vi "WS1050 Bench CAP Characterization_Ver1.1.vi"() -> ()   [LabVIEW 2012]
panel:
  in  "Tab Control":enum32{"CONTROL", "INDICATION"}(tab)
  in  "RFFE Com Port":refnum<visa-resource-name>="COM3"
  in  "AD7747 Com Port":refnum<visa-resource-name>="COM1"
  in  "Init":bool=TRUE
  in  "Wafer":string="WS1050"
  in  "Lot":string="Toggle 7"
  in  "SN":string="01"
  in  "Temperature":string="RT"
  in  "Delay(ms)":u32=100
  in  "TMN DC\\CAP Data Log File Path":path=path "C:/Andy Tr/Temp"
  in  "String":string="WS1050 BENCH CAP CHARACTERIZATION Ver1.1"
  out "C3Cal (pF)":dbl=-4.9974111328125
  out "C1Cal (pF)":dbl=-4.5642919921875
  out "C2Cal (pF)":dbl=-4.9191376953125
  out "S_ValueC3(pF)":dbl=-4.9974111328125
  out "S_ValueC1(pF)":dbl=-4.5642919921875
  out "S_ValueC2(pF)":dbl=-4.9191376953125
  in  "Calib Socket":bool
  out "C1_Mesa(pF)":dbl
  out "C2_Mesa(pF)":dbl
  out "C3_Mesa(pF)":dbl
  in  "A364X_VDD":refnum<visa-resource-name>="GPIB1::6::INSTR"
  in  "IDD Limit":dbl=0.02 format="%.2p"
  in  "VDD":dbl=3.3
  in  "CP Setting":i32(ring) items=["CP OFF", "CP ON", "DVA OFF", "DVA ON", "ECAL OFF", "ECAL ON", "CP 40.25V", "CP 35V", "CP 38V", "CP 44V", "CP 50V", "CP 23.75V", "CP 25.25V", "CP 29.75V", "C1 ON", "C1 OFF", "C2 ON", "C2 OFF", "C3 ON", "C3 OFF"]
  in  "Send":bool
  in  "Init AD7747":bool
  in  "Keithley 2000":refnum<visa-resource-name>
  out "C_min(pF)":string[](array[string])
  out "C_Max":string[](array[string])
  out "C_Min2(pF)":string[](array[string])
  out "error out":errorcluster
  in  "error in (no error)":errorcluster
  in  "stop":bool
  in  "Abort":bool
  in  "Start Test":bool
  out "Running loop":i32
  # "Company:  WiSpry Inc\n198 Fairbanks Ste 198 Irvine\n\nCreated by:  Andy V Tran\nDate:  03/11/2015\nTP:  WS1050 Bench\nCAP Characterization"
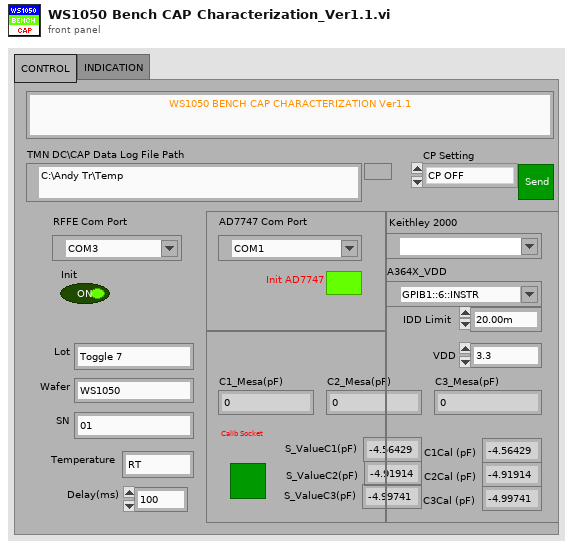
[diagram p1: front panel]
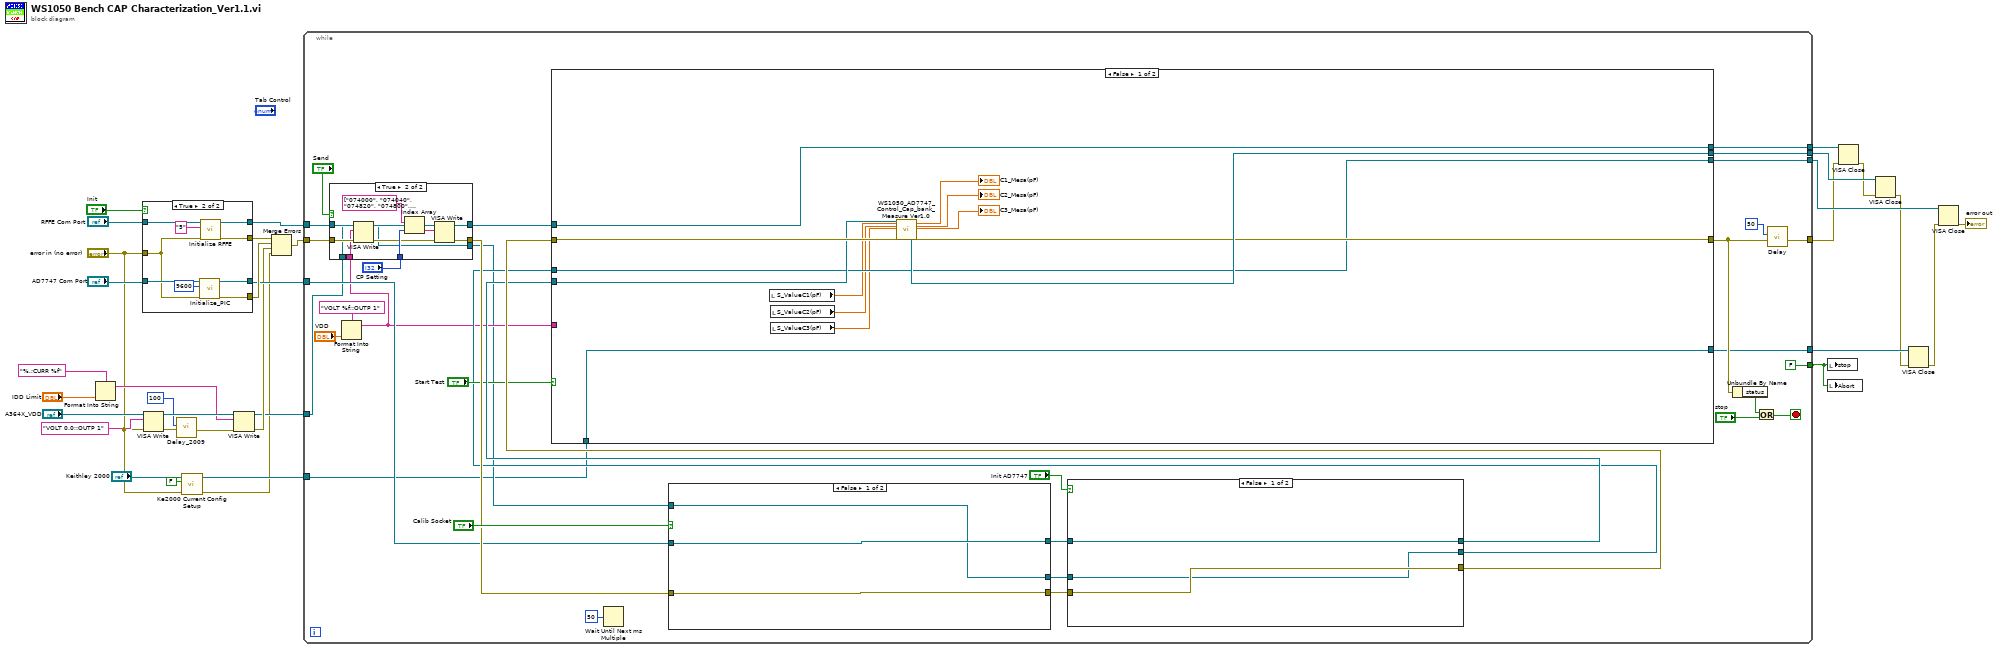
[diagram p0: block diagram]
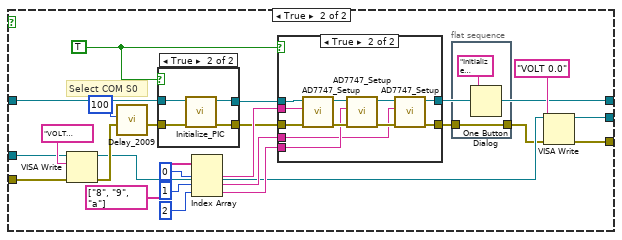
[diagram p3: hidden frame]
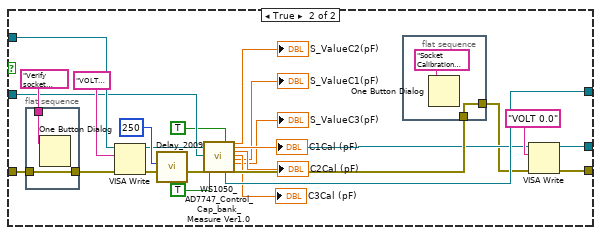
[diagram p6: hidden frame]
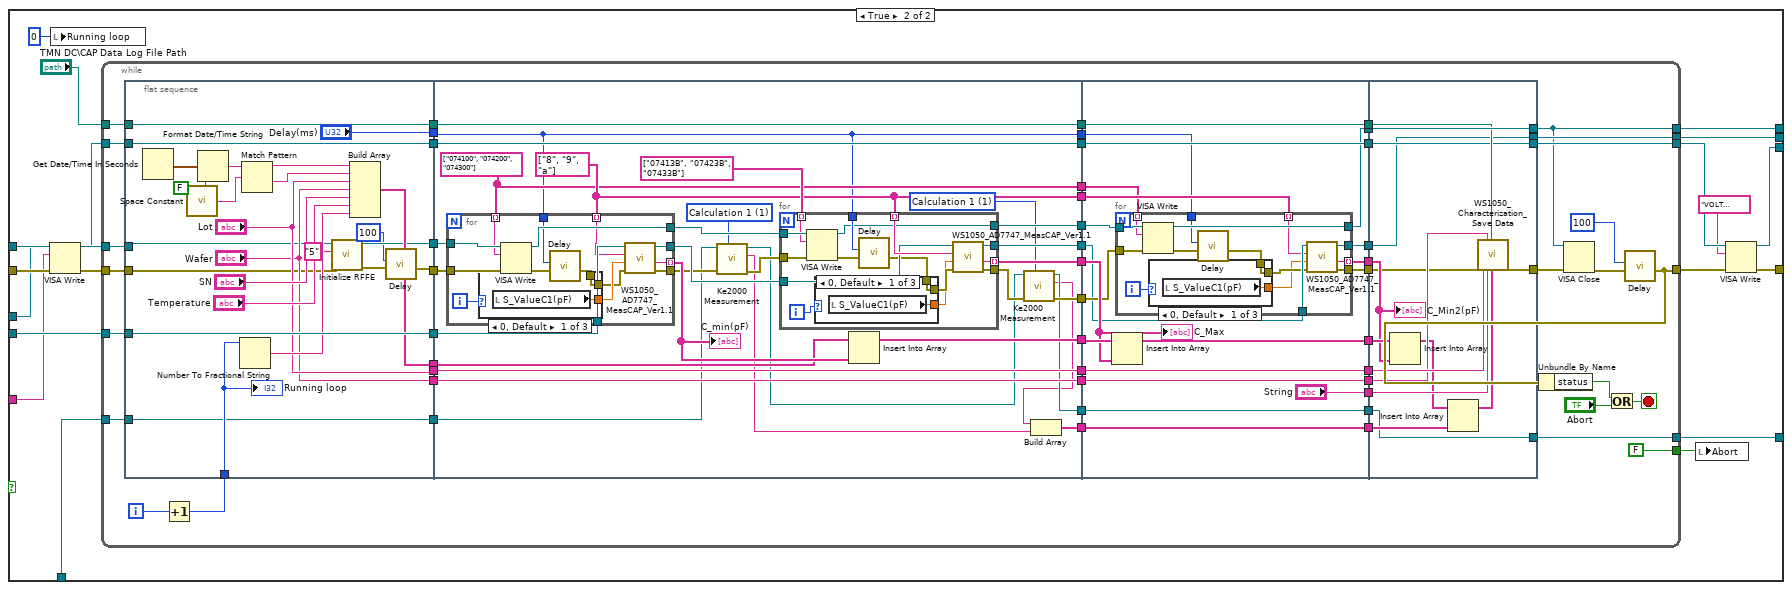
[diagram p7: hidden frame]
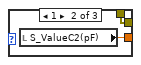
[diagram p8: hidden frame]
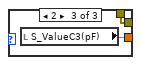
[diagram p9: hidden frame]
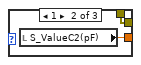
[diagram p10: hidden frame]
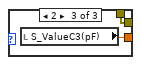
[diagram p11: hidden frame]
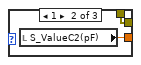
[diagram p12: hidden frame]
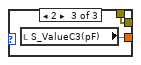
[diagram p13: hidden frame]
diagram:
  n1 = Format Into String(format string="%.;CURR %f", "IDD Limit") -> (resulting string=w24:string)  [unwired: 2 in, 1 out]
  n2 = case shown="True" "Init" {
    tunnel: "RFFE Com Port" -> [w37 w46]
    tunnel: [w37 w44] -> w33
    tunnel: "AD7747 Com Port" -> [w35 w42]
    tunnel: [w36 w41] -> w31
    tunnel: [w36 w40] -> w30
    tunnel: [w35 w39] -> w28
    tunnel: "error in (no error)" -> [w36 w38]
    frame False {
    }
    frame True {
      n3 = call "Initialize_PIC.vi"("error in (no error)"=w38, "baud rate"=u32 9600, "Select Com Port"=w42) -> ("error out"=w40:errorcluster, "VISA resource name out"=w39:refnum<visa-resource-name>)  [unwired: 7 in]
      n4 = call "Initialize RFFE.vi"("error in (no error)"=w38, "write buffer"="5", "Select Com Port"=w46) -> ("error out"=w41:errorcluster, "VISA resource name out"=w44:refnum<visa-resource-name>)  [unwired: 7 in]
    }
  }
  n5 = VISA Write(VISA resource name="A364X_VDD", write buffer="VOLT 0.0;:OUTP 1", error in (no error)="error in (no error)") -> (VISA resource name out=w25:refnum<visa-resource-name>, error out=w21:errorcluster)  [unwired: 1 out]
  n6 = call "Delay_2009.vi"("error in (no error)"=w21, "milliseconds to wait"=u32 100) -> ("error out"=w26:errorcluster)  [unwired: 9 in]
  n7 = call "Ke2000 Current Config Setup.vi"("error in (no error)"="error in (no error)", "Auto Range(T/F)"=FALSE, "VISA resource name"="Keithley 2000") -> ("error out"=w4:errorcluster, "VISA resource name out"=w5:refnum<visa-resource-name>)  [unwired: 7 in]
  n8 = VISA Write(VISA resource name=w25, write buffer=w24, error in (no error)=w26) -> (VISA resource name out=w16:refnum<visa-resource-name>, error out=w17:errorcluster)  [unwired: 1 out]
  n9 = Merge Errors(w31, w30, w17, w4) -> (w29:errorcluster)
  n10 = while {
    tunnel: w33 -> [w77]
    tunnel: w29 -> [w78]
    tunnel: w28 -> [w65]
    tunnel: [w73] -> w12
    tunnel: [w71] -> w15
    tunnel: [w70] -> w14
    tunnel: w16 -> [w52]
    tunnel: [w56] -> w13
    tunnel: [FALSE ("stop")] -> w9
    tunnel: w5 -> [w48]
    tunnel: [w47] -> w3
    stop <- w68 stop-if-true
    n11 = Format Into String(format string="VOLT %f;:OUTP 1", "VDD") -> (resulting string=w51:string)  [unwired: 2 in, 1 out]
    n12 = case shown="True" "Send" {
      tunnel: w78 -> [w404 w410]
      tunnel: [w404 w414] -> w66
      tunnel: [w403 w413] -> w76
      tunnel: "CP Setting" -> [_ w412]
      tunnel: w77 -> [w403 w411]
      tunnel: w52 -> [w402 w409]
      tunnel: w51 -> [_ w408]
      tunnel: [w402 w406] -> w50
      frame False {
      }
      frame True {
        n13 = VISA Write(VISA resource name=w409, write buffer=w408, error in (no error)=w410) -> (VISA resource name out=w406:refnum<visa-resource-name>, error out=w407:errorcluster)  [unwired: 1 out]
        n14 = Index Array(array=string[] ["074000", "074040", "074820", "074800", "074044", "074040", "074776", "07476F", "074773", "07477B", "07477C", "074760", "074762", "074768", "07413B", "074100", "07423B", "074200", "07433B", "074300"], index=w412) -> (element=w415:string)
        n15 = VISA Write(VISA resource name=w411, write buffer=w415, error in (no error)=w407) -> (VISA resource name out=w413:refnum<visa-resource-name>, error out=w414:errorcluster)  [unwired: 1 out]
      }
    }
    n16 = Wait Until Next ms Multiple(millisecond multiple=u32 50) -> ()  [unwired: 1 out]
    n17 = case shown="False" "Calib Socket" {
      tunnel: w66 -> [w131 w154]
      tunnel: [w131 w137] -> w60
      tunnel: w65 -> [w130 w135]
      tunnel: w50 -> [w129 w143]
      tunnel: [w129 w138] -> w61
      tunnel: [w130 w152] -> w59
      frame False {
      }
      frame True {
        n18 = flat-sequence {
          tunnel: [w157] -> w144
          tunnel: w154 -> [w157]
          tunnel: "Verify socket should be empty" ("message") -> [w156]
          frame #0 {
            n19 = One Button Dialog(message=w156) -> ()  [unwired: 1 in, 1 out]
          }
        }
        n20 = VISA Write(VISA resource name=w143, write buffer="VOLT 3.3;:OUTP 1", error in (no error)=w144) -> (VISA resource name out=w139:refnum<visa-resource-name>, error out=w141:errorcluster)  [unwired: 1 out]
        n21 = call "Delay_2009.vi"("error in (no error)"=w141, "milliseconds to wait"=u32 250) -> ("error out"=w134:errorcluster)  [unwired: 9 in]
        n22 = call "WS1050_AD7747_Control_Cap_bank_Measure Ver1.0.vi"("Select Com Port"=w135, "errorin"=w134, "Push Button to Measue Cap"=TRUE, "Push Button to Calibrate"=TRUE ("Push Button to Initialize AD7747")) -> ("Com Port Out"=w152:refnum<visa-resource-name>, "C2(pF)"=→"S_ValueC2(pF)":dbl, "C1_Mesa(pF)"=→"C1Cal (pF)":dbl, "C2_Mesa(pF)"=→"C2Cal (pF)":dbl, "C3_Mesa(pF)"=→"C3Cal (pF)":dbl, "C1(pF)"=→"S_ValueC1(pF)":dbl, "C3(pF)"=→"S_ValueC3(pF)":dbl, "error out"=w153:errorcluster)  [unwired: 16 in]
        n23 = flat-sequence {
          tunnel: [w158] -> w136
          tunnel: w153 -> [w158]
          frame #0 {
            n24 = One Button Dialog(message="Socket Calibration Completed, Please insert DUT into the Socket") -> ()  [unwired: 1 in, 1 out]
          }
        }
        n25 = VISA Write(VISA resource name=w139, write buffer="VOLT 0.0", error in (no error)=w136) -> (VISA resource name out=w138:refnum<visa-resource-name>, error out=w137:errorcluster)  [unwired: 1 out]
      }
    }
    n26 = case shown="False" "Init AD7747" {
      tunnel: w59 -> [w82 w107]
      tunnel: [w83 w87] -> w63
      tunnel: w60 -> [w83 w92]
      tunnel: [w82 w85] -> w62
      tunnel: w61 -> [w81 w93]
      tunnel: [w81 w88] -> w57
      frame False {
      }
      frame True {
        w97 = TRUE
        # "Select COM S0"
        n27 = VISA Write(VISA resource name=w93, write buffer="VOLT 3.3;:OUTP 1", error in (no error)=w92) -> (VISA resource name out=w89:refnum<visa-resource-name>, error out=w91:errorcluster)  [unwired: 1 out]
        n28 = call "Delay_2009.vi"("error in (no error)"=w91, "milliseconds to wait"=u32 100) -> ("error out"=w95:errorcluster)  [unwired: 9 in]
        n29 = case shown="True" w97 {
          tunnel: [w121 w126] -> w98
          tunnel: [w122 w125] -> w106
          tunnel: w107 -> [w122 w124]
          tunnel: w95 -> [w121 w123]
          frame False {
          }
          frame True {
            n30 = call "Initialize_PIC.vi"("error in (no error)"=w123, "Select Com Port"=w124) -> ("error out"=w126:errorcluster, "VISA resource name out"=w125:refnum<visa-resource-name>)  [unwired: 8 in]
          }
        }
        n31 = Index Array(array=string[] ["8", "9", "a"], index #1=0 ("index"), index #2=1 ("index"), index #3=2 ("index")) -> (element #1=w101:string, element #2=w100:string, element #3=w99:string)
        n32 = case shown="True" w97 {
          tunnel: w98 -> [w109 w112]
          tunnel: [w109 w110] -> w84
          tunnel: w106 -> [w108 w120]
          tunnel: w101 -> [_ w115]
          tunnel: w99 -> [_ w114]
          tunnel: w100 -> [_ w113]
          tunnel: [w108 w111] -> w85
          frame False {
          }
          frame True {
            n33 = call "AD7747_Setup.vi"("error in"=w112, "AD7747_Number"=w115, "Control"=w120) -> ("error out"=w119:errorcluster, "Control out"=w118:refnum<visa-resource-name>)  [unwired: 6 in, 1 out]
            n34 = call "AD7747_Setup.vi"("error in"=w119, "AD7747_Number"=w114, "Control"=w118) -> ("error out"=w117:errorcluster, "Control out"=w116:refnum<visa-resource-name>)  [unwired: 6 in, 1 out]
            n35 = call "AD7747_Setup.vi"("error in"=w117, "AD7747_Number"=w113, "Control"=w116) -> ("error out"=w110:errorcluster, "Control out"=w111:refnum<visa-resource-name>)  [unwired: 6 in, 1 out]
          }
        }
        n36 = flat-sequence {
          tunnel: w84 -> [w127]
          tunnel: [w127] -> w86
          frame #0 {
            n37 = One Button Dialog(message="Initialize AD7747 completed!") -> ()  [unwired: 1 in, 1 out]
          }
        }
        n38 = VISA Write(VISA resource name=w89, write buffer="VOLT 0.0", error in (no error)=w86) -> (VISA resource name out=w88:refnum<visa-resource-name>, error out=w87:errorcluster)  [unwired: 1 out]
      }
    }
    n39 = case shown="False" "Start Test" {
      tunnel: w76 -> [w165 w191]
      tunnel: w63 -> [w172 w186]
      tunnel: w62 -> [w171 w190]
      tunnel: [w169 w184] -> w74
      tunnel: [w165 w189] -> w71
      tunnel: [w170 w188] -> w70
      tunnel: w57 -> [w164 w185]
      tunnel: [w164 w181] -> w56
      tunnel: w51 -> [_ w176]
      tunnel: w48 -> [w160 w174]
      tunnel: [w160 w173] -> w47
      frame False {
        n40 = local read "S_ValueC1(pF)"() -> (w163:dbl)
        n41 = local read "S_ValueC2(pF)"() -> (w162:dbl)
        n42 = local read "S_ValueC3(pF)"() -> (w161:dbl)
        n43 = call "WS1050_AD7747_Control_Cap_bank_Measure Ver1.0.vi"("Select Com Port"=w171, "S_Value C1"=w163, "S_Value C2"=w162, "S_Value C3"=w161, "errorin"=w172) -> ("Com Port Out"=w170:refnum<visa-resource-name>, "C1_Mesa(pF)"=→"C1_Mesa(pF)":dbl, "C2_Mesa(pF)"=→"C2_Mesa(pF)":dbl, "C3_Mesa(pF)"=→"C3_Mesa(pF)":dbl, "error out"=w169:errorcluster)  [unwired: 15 in, 3 out]
      }
      frame True {
        n44 = VISA Write(VISA resource name=w185, write buffer=w176, error in (no error)=w186) -> (VISA resource name out=w183:refnum<visa-resource-name>, error out=w187:errorcluster)  [unwired: 1 out]
        n45 = local write "Running loop"(0 ("Loop Running")) -> ()
        n46 = while {
          tunnel: w191 -> [w244]
          tunnel: w187 -> [w243]
          tunnel: w190 -> [w242]
          tunnel: [w199] -> w180
          tunnel: "TMN DC\\CAP Data Log File Path" -> [w236]
          tunnel: [w202] -> w189
          tunnel: [w232] -> w188
          tunnel: w183 -> [w228]
          tunnel: [w225] -> w182
          tunnel: [FALSE ("Abort")] -> w177
          tunnel: w174 -> [w198]
          tunnel: [w192] -> w173
          i -> [w219]
          stop <- w239 stop-if-true
          n47 = flat-sequence {
            tunnel: w228 -> [w270]
            tunnel: w236 -> [w271]
            tunnel: w242 -> [w272]
            tunnel: w243 -> [w253]
            tunnel: w244 -> [w254]
            tunnel: [w250] -> w217
            tunnel: [w251] -> w216
            tunnel: [w272] -> w215
            tunnel: [w271] -> w214
            tunnel: [w270] -> w213
            tunnel: w212 -> [w257]
            tunnel: [w260] -> w211
            tunnel: ["Lot"] -> w210
            tunnel: ["Wafer"] -> w207
            tunnel: ["Delay(ms)"] -> w203
            tunnel: w198 -> [w248]
            tunnel: [w248] -> w197
            tunnel: [w292] -> w247
            tunnel: [w297] -> w246
            tunnel: [w279] -> w241
            tunnel: [w296] -> w235
            tunnel: [w295] -> w233
            tunnel: [w294] -> w230
            tunnel: [w291] -> w226
            tunnel: [w290] -> w224
            tunnel: [w285] -> w223
            tunnel: [w289] -> w222
            tunnel: w217 -> [w303]
            tunnel: w216 -> [w302]
            tunnel: w215 -> [w299]
            tunnel: w214 -> [w294]
            tunnel: w213 -> [w291]
            tunnel: w211 -> [w288]
            tunnel: w210 -> [w287]
            tunnel: [w287] -> w209
            tunnel: w207 -> [w286]
            tunnel: [w286] -> w206
            tunnel: w203 -> [w285]
            tunnel: w197 -> [w282]
            tunnel: [w277] -> w196
            tunnel: [w273] -> w194
            tunnel: w247 -> [w365]
            tunnel: w246 -> [w364]
            tunnel: [w363] -> w245
            tunnel: w241 -> [w359]
            tunnel: [w360] -> w240
            tunnel: w235 -> [w355]
            tunnel: [w354] -> w234
            tunnel: w233 -> [w353]
            tunnel: [w362] -> w231
            tunnel: w230 -> [w362]
            tunnel: [w361] -> w227
            tunnel: w226 -> [w361]
            tunnel: w224 -> [w358]
            tunnel: w223 -> [w357]
            tunnel: w222 -> [w356]
            tunnel: [w352] -> w221
            tunnel: [w351] -> w220
            tunnel: w209 -> [w350]
            tunnel: [w350] -> w208
            tunnel: w206 -> [w349]
            tunnel: [w349] -> w205
            tunnel: ["String"] -> w204
            tunnel: w196 -> [w347]
            tunnel: [w347] -> w195
            tunnel: w194 -> [w346]
            tunnel: [w346] -> w193
            tunnel: w245 -> [w396]
            tunnel: w240 -> [w391]
            tunnel: [w401] -> w201
            tunnel: w234 -> [w400]
            tunnel: [w400] -> w202
            tunnel: [w397] -> w232
            tunnel: w231 -> [w399]
            tunnel: w227 -> [w398]
            tunnel: [w398] -> w225
            tunnel: w221 -> [w397]
            tunnel: w220 -> [w395]
            tunnel: w208 -> [w394]
            tunnel: w205 -> [w393]
            tunnel: w204 -> [w392]
            tunnel: w195 -> [w387]
            tunnel: w193 -> [w389]
            tunnel: [w387] -> w192
            frame #0 {
              n48 = Get Date/Time In Seconds() -> (seconds since 1Jan1904=w266:timestamp)
              n49 = call <vilib>:"Space Constant.vi"() -> ("String"=w269:string)
              n50 = Format Date/Time String(seconds (now)=w266, UTC format=FALSE) -> (date/time string=w267:string)  [unwired: 1 out]
              n51 = Number To Fractional String(number=w257) -> (F-format string=w261:string)  [unwired: 3 in]
              n52 = Match Pattern(string=w267, regular expression=w269) -> (before substring=w265:string, after substring=w264:string)  [unwired: 3 out]
              n53 = call "Initialize RFFE.vi"("error in (no error)"=w253, "write buffer"="5", "Select Com Port"=w254) -> ("error out"=w252:errorcluster, "VISA resource name out"=w250:refnum<visa-resource-name>)  [unwired: 7 in]
              n54 = Build Array(w265, w264, "Lot", "Wafer", "SN", "Temperature", w261) -> (w260:string[])
              n55 = call "Delay.vi"("error in (no error)"=w252, "milliseconds to wait"=u32 100) -> ("error out"=w251:errorcluster)  [unwired: 9 in]
              "Running loop" <- w257
            }
            frame #1 {
              w276 = u16 1 items=["Function", "Calculation 1", "Calculation 2", "Calculation 3"] ("Source (0: Function)")
              w281 = u16 1 items=["Function", "Calculation 1", "Calculation 2", "Calculation 3"] ("Source (0: Function)")
              w290 = string[] ["8", "9", "a"]
              w289 = string[] ["074100", "074200", "074300"]
              n56 = for {
                tunnel: w303 -> [w339]
                tunnel: w302 -> [w338]
                tunnel: w289 -> [w337] mode=indexing
                tunnel: [w336] -> w300
                tunnel: w299 -> [w335]
                tunnel: [w334] -> w298
                tunnel: [w333] -> w283
                tunnel: w285 -> [w331]
                tunnel: w290 -> [w330] mode=indexing
                tunnel: [w329] -> w293 mode=indexing
                i -> [w328]
                n57 = VISA Write(VISA resource name=w339, write buffer=w337, error in (no error)=w338) -> (VISA resource name out=w336:refnum<visa-resource-name>, error out=w332:errorcluster)  [unwired: 1 out]
                n58 = call "Delay.vi"("error in (no error)"=w332, "milliseconds to wait"=w331) -> ("error out"=w326:errorcluster)  [unwired: 9 in]
                n59 = case shown="0, Default" w328 {
                  tunnel: [w341 w343 w345] -> w327
                  tunnel: w326 -> [w340 w342 w344]
                  tunnel: [w340 w342 w344] -> w325
                  frame 0, Default {
                    n60 = local read "S_ValueC1(pF)"() -> (w341:dbl)
                  }
                  frame 1 {
                    n61 = local read "S_ValueC2(pF)"() -> (w343:dbl)
                  }
                  frame 2 {
                    n62 = local read "S_ValueC3(pF)"() -> (w345:dbl)
                  }
                }
                n63 = call "WS1050_AD7747_MeasCAP_Ver1.1.vi"("error in (no error)"=w325, "OFFSet Cal"=w327, "AD7747_Number"=w330, "Control"=w335) -> ("error"=w333:errorcluster, "CAP (pF)"=w329:string, "Control out"=w334:refnum<visa-resource-name>)  [unwired: 4 in, 1 out]
              }
              "C_min(pF)" <- w293
              n64 = call "Ke2000 Measurement.vi"("Source (0: Function)"=w281, "error in (no error)"=w283, "VISA resource name"=w282) -> ("error out"=w284:errorcluster, "Meas in micro"=w274:string, "VISA resource name out"=w278:refnum<visa-resource-name>)  [unwired: 3 in, 3 out]
              n65 = for {
                tunnel: w300 -> [w318]
                tunnel: w284 -> [w317]
                tunnel: string[] ["07413B", "07423B", "07433B"] -> [w316] mode=indexing
                tunnel: w285 -> [w314]
                tunnel: w290 -> [w313] mode=indexing
                tunnel: [w312] -> w280
                tunnel: [w311] -> w295
                tunnel: [w310] -> w296
                tunnel: w298 -> [w309]
                tunnel: [w308] -> w297 mode=indexing
                i -> [w306]
                n66 = VISA Write(VISA resource name=w318, write buffer=w316, error in (no error)=w317) -> (VISA resource name out=w310:refnum<visa-resource-name>, error out=w315:errorcluster)  [unwired: 1 out]
                n67 = call "Delay.vi"("error in (no error)"=w315, "milliseconds to wait"=w314) -> ("error out"=w305:errorcluster)  [unwired: 9 in]
                n68 = case shown="0, Default" w306 {
                  tunnel: [w320 w322 w324] -> w304
                  tunnel: w305 -> [w319 w321 w323]
                  tunnel: [w319 w321 w323] -> w307
                  frame 0, Default {
                    n69 = local read "S_ValueC1(pF)"() -> (w320:dbl)
                  }
                  frame 1 {
                    n70 = local read "S_ValueC2(pF)"() -> (w322:dbl)
                  }
                  frame 2 {
                    n71 = local read "S_ValueC3(pF)"() -> (w324:dbl)
                  }
                }
                n72 = call "WS1050_AD7747_MeasCAP_Ver1.1.vi"("error in (no error)"=w307, "OFFSet Cal"=w304, "AD7747_Number"=w313, "Control"=w309) -> ("error"=w312:errorcluster, "CAP (pF)"=w308:string, "Control out"=w311:refnum<visa-resource-name>)  [unwired: 4 in, 1 out]
              }
              n73 = Insert Into Array(array=w288, new element=w293) -> (w292:string[])  [unwired: 1 in]
              n74 = call "Ke2000 Measurement.vi"("Source (0: Function)"=w276, "error in (no error)"=w280, "VISA resource name"=w278) -> ("error out"=w279:errorcluster, "Meas in micro"=w275:string, "VISA resource name out"=w277:refnum<visa-resource-name>)  [unwired: 3 in, 3 out]
              n75 = Build Array(w275, w274) -> (w273:string[])
            }
            frame #2 {
              n76 = Insert Into Array(array=w365, new element=w364) -> (w363:string[])  [unwired: 1 in]
              n77 = for {
                tunnel: w355 -> [w380]
                tunnel: w359 -> [w379]
                tunnel: w356 -> [w378] mode=indexing
                tunnel: [w377] -> w354
                tunnel: w353 -> [w376]
                tunnel: [w375] -> w352
                tunnel: [w374] -> w360
                tunnel: w357 -> [w372]
                tunnel: w358 -> [w371] mode=indexing
                tunnel: [w370] -> w351 mode=indexing
                i -> [w369]
                n78 = VISA Write(VISA resource name=w380, write buffer=w378, error in (no error)=w379) -> (VISA resource name out=w377:refnum<visa-resource-name>, error out=w373:errorcluster)  [unwired: 1 out]
                n79 = call "Delay.vi"("error in (no error)"=w373, "milliseconds to wait"=w372) -> ("error out"=w367:errorcluster)  [unwired: 9 in]
                n80 = case shown="0, Default" w369 {
                  tunnel: [w382 w384 w386] -> w366
                  tunnel: w367 -> [w381 w383 w385]
                  tunnel: [w381 w383 w385] -> w368
                  frame 0, Default {
                    n81 = local read "S_ValueC1(pF)"() -> (w382:dbl)
                  }
                  frame 1 {
                    n82 = local read "S_ValueC2(pF)"() -> (w384:dbl)
                  }
                  frame 2 {
                    n83 = local read "S_ValueC3(pF)"() -> (w386:dbl)
                  }
                }
                n84 = call "WS1050_AD7747_MeasCAP_Ver1.1.vi"("error in (no error)"=w368, "OFFSet Cal"=w366, "AD7747_Number"=w371, "Control"=w376) -> ("error"=w374:errorcluster, "CAP (pF)"=w370:string, "Control out"=w375:refnum<visa-resource-name>)  [unwired: 4 in, 1 out]
              }
              "C_Max" <- w364
            }
            frame #3 {
              n85 = Insert Into Array(array=w396, new element=w395) -> (w390:string[])  [unwired: 1 in]
              n86 = Insert Into Array(array=w390, new element=w389) -> (w388:string[])  [unwired: 1 in]
              n87 = call "WS1050_Characterization_Save Data.vi"("error in (no error)"=w391, "Lot"=w394, "Wafer"=w393, "TP"=w392, "TMN DC\\CAP Data Log File Path"=w399, "All Out"=w388) -> ("error out"=w401:errorcluster)  [unwired: 19 in, 2 out]
              "C_Min2(pF)" <- w395
            }
          }
          n88 = Increment(x=w219) -> (x+1=w212:i32)
          n89 = VISA Close(VISA resource name=w202, error in (no error)=w201) -> (error out=w200:errorcluster)
          n90 = call "Delay.vi"("error in (no error)"=w200, "milliseconds to wait"=u32 100) -> ("error out"=w199:errorcluster)  [unwired: 9 in]
          n91 = Unbundle By Name(w199) -> ("status"=w238:bool)
          n92 = Or(x=w238, y="Abort") -> (x .or. y?=w239:bool)
        }
        n93 = local write "Abort"(w177) -> ()
        n94 = VISA Write(VISA resource name=w182, write buffer="VOLT 0.0;:OUTP 0", error in (no error)=w180) -> (VISA resource name out=w181:refnum<visa-resource-name>, error out=w184:errorcluster)  [unwired: 1 out]
      }
    }
    n95 = Unbundle By Name(w74) -> ("status"=w75:bool)
    n96 = Or(x=w75, y="stop") -> (x .or. y?=w68:bool)
    n97 = call "Delay.vi"("error in (no error)"=w74, "milliseconds to wait"=u32 50) -> ("error out"=w73:errorcluster)  [unwired: 9 in]
  }
  n98 = local write "stop"(w9) -> ()
  n99 = local write "Abort"(w9) -> ()
  n100 = VISA Close(VISA resource name=w15, error in (no error)=w12) -> (error out=w11:errorcluster)
  n101 = VISA Close(VISA resource name=w14, error in (no error)=w11) -> (error out=w2:errorcluster)
  n102 = VISA Close(VISA resource name=w3, error in (no error)=w2) -> (error out=w1:errorcluster)
  n103 = VISA Close(VISA resource name=w13, error in (no error)=w1) -> (error out=→"error out":errorcluster)
